vi "initialize.vi"(8 "error in (no error)":errorcluster, 11 "Camera in":refnum<class "Camera.lvclass">) -> (0 "error out":errorcluster, 3 "Camera out":refnum<class "Camera.lvclass">)   [LabVIEW 2013, in "Camera.lvclass"]
uses:
  Camera.lvclass
  Camera.lvclass/Camera.ctl
  Experiment/Globals.vi
panel:
  in  "shots per measurement":i32
  in  "Use camera?":bool
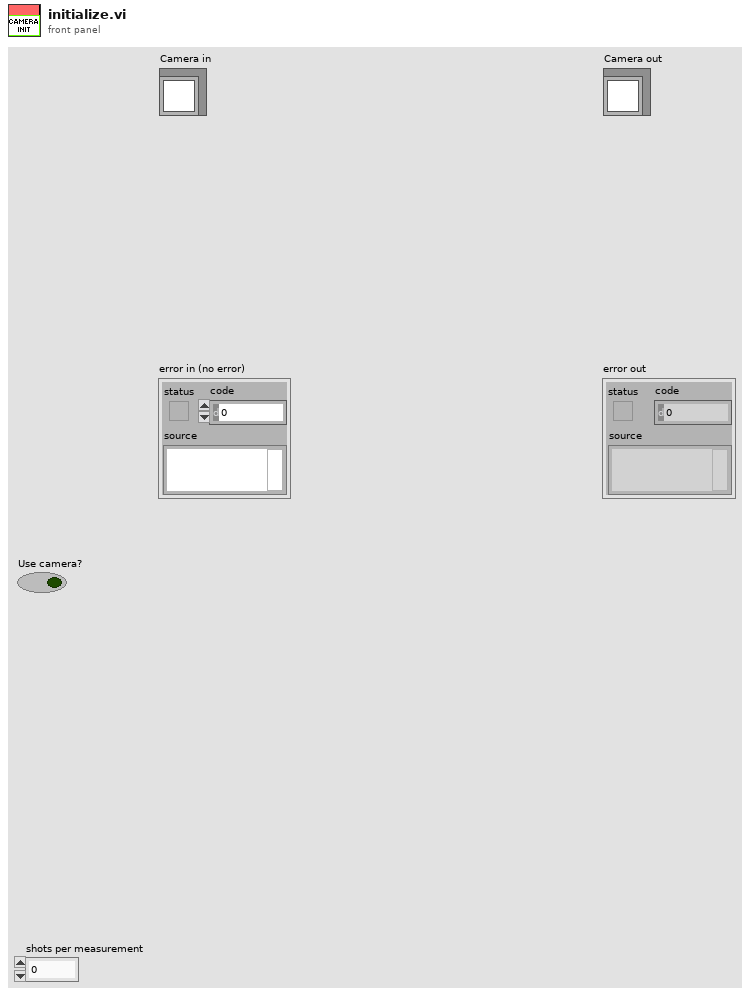
[diagram p1: front panel]
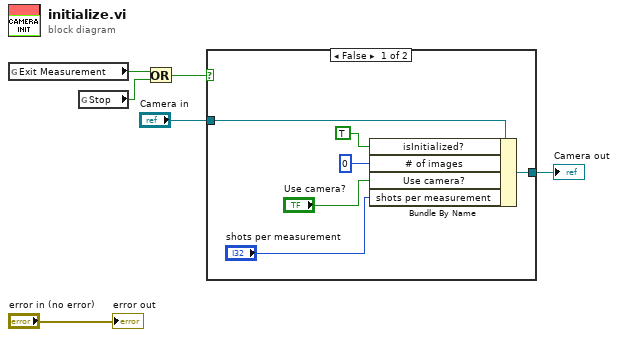
[diagram p0: block diagram]
diagram:
  n1 = global read "Globals.vi" "Exit Measurement"() -> (w2:bool)
  n2 = global read "Globals.vi" "Stop"() -> (w3:bool)
  n3 = Or(x=w2, y=w3) -> (x .or. y?=w1:bool)
  n4 = case shown="False" w1 {
    tunnel: "Camera in" -> [w12 w13]
    tunnel: [w11 w13] -> w4
    frame False {
      n5 = Bundle By Name(cluster=w12, "isInitialized?"=TRUE, "# of images"=u32 0, "Use camera?"="Use camera?", "shots per measurement"="shots per measurement") -> (w11:refnum<class "Camera.lvclass">)
    }
    frame True {
    }
  }
  "Camera out" <- w4
  "error out" <- "error in (no error)"
